vi "Main.vi"() -> ()   [LabVIEW 2013]
uses:
  <vilib>/myRIO/Instrument Drivers/Onboard IO/I2C/vis/Smart Open.vi
  <vilib>/myRIO/Instrument Drivers/Onboard IO/I2C/vis/Configure.vi
  <vilib>/myRIO/Instrument Drivers/Onboard IO/I2C/vis/Write.vi
  <vilib>/myRIO/Common/Instrument Driver Framework/myRIO v1.0/UART/vis/myRIO v1.0 Close UART.vi
  <vilib>/myRIO/Instrument Drivers/Onboard IO/I2C/vis/Open.vi
  <vilib>/myRIO/Common/Instrument Driver Framework/myRIO v1.0/I2C/vis/myRIO v1.1 Open I2C.vi
  <vilib>/myRIO/Common/Instrument Driver Framework/Utilities/vis/Validate Channels.vi
  <vilib>/myRIO/Common/Instrument Driver Framework/myRIO v1.0/I2C/vis/myRIO v1.0 Reserve I2C.vi
  <vilib>/myRIO/Common/Instrument Driver Framework/myRIO v1.0/I2C/vis/myRIO v1.0 Build MUX Configuration I2C.vi
  <vilib>/myRIO/Common/Instrument Driver Framework/myRIO v1.0/Resource Manager/vis/myRIO v1.0 Reserve Channel List.vi
  <vilib>/myRIO/Common/Instrument Driver Framework/myRIO v1.0/Resource Manager/vis/myRIO v1.0 Create Configuration List.vi
  <vilib>/myRIO/Common/Instrument Driver Framework/myRIO v1.0/Resource Manager/vis/myRIO v1.0 Reserve Channel.vi
  <vilib>/myRIO/Common/Instrument Driver Framework/myRIO v1.0/Resource Manager/vis/myRIO v1.0 Unreserve Channel.vi
  <vilib>/myRIO/Common/Instrument Driver Framework/myRIO v1.0/Resource Manager/vis/myRIO v1.0 Build Mutex Name.vi
  <vilib>/Instr/_visa.llb/VISA Configure Serial Port (Instr).vi
  <vilib>/myRIO/Common/Instrument Driver Framework/myRIO v1.0/myRIO v1.1 Open.vi
  <vilib>/Utility/VariantDataType/GetNumericInfo.vi
  <vilib>/Utility/error.llb/Error Cluster From Error Code.vi
  <vilib>/myRIO/Common/Instrument Driver Framework/Utilities/vis/IO Manager.vi
  <vilib>/myRIO/Common/Instrument Driver Framework/Utilities/vis/Configuration Manager.vi
  <vilib>/myRIO/Common/Instrument Driver Framework/myRIO v1.0/Resource Manager/vis/myRIO v1.0 Configure IO.vi
  <vilib>/myRIO/Common/Instrument Driver Framework/myRIO v1.0/myRIO v1.0 Close.vi
  <vilib>/myRIO/Common/Instrument Driver Framework/myRIO v1.0/I2C/vis/myRIO v1.0 Configure I2C.vi
  <vilib>/myRIO/Common/Instrument Driver Framework/myRIO v1.0/I2C/vis/myRIO v1.0 Write I2C.vi
  <vilib>/myRIO/Common/Instrument Driver Framework/Utilities/vis/FPGA Ref Manager.vi
  <vilib>/myRIO/Common/Instrument Driver Framework/myRIO v1.0/myRIO v1.0 Reset FPGA.vi
  <vilib>/myRIO/Instrument Drivers/Utilities/Utilities.lvlib
panel:
  in  "[ESC]":bool
  # "Digital tape measure"
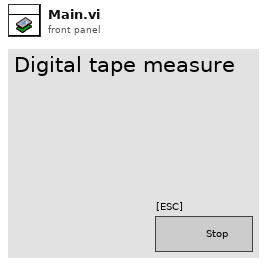
[diagram p1: front panel]
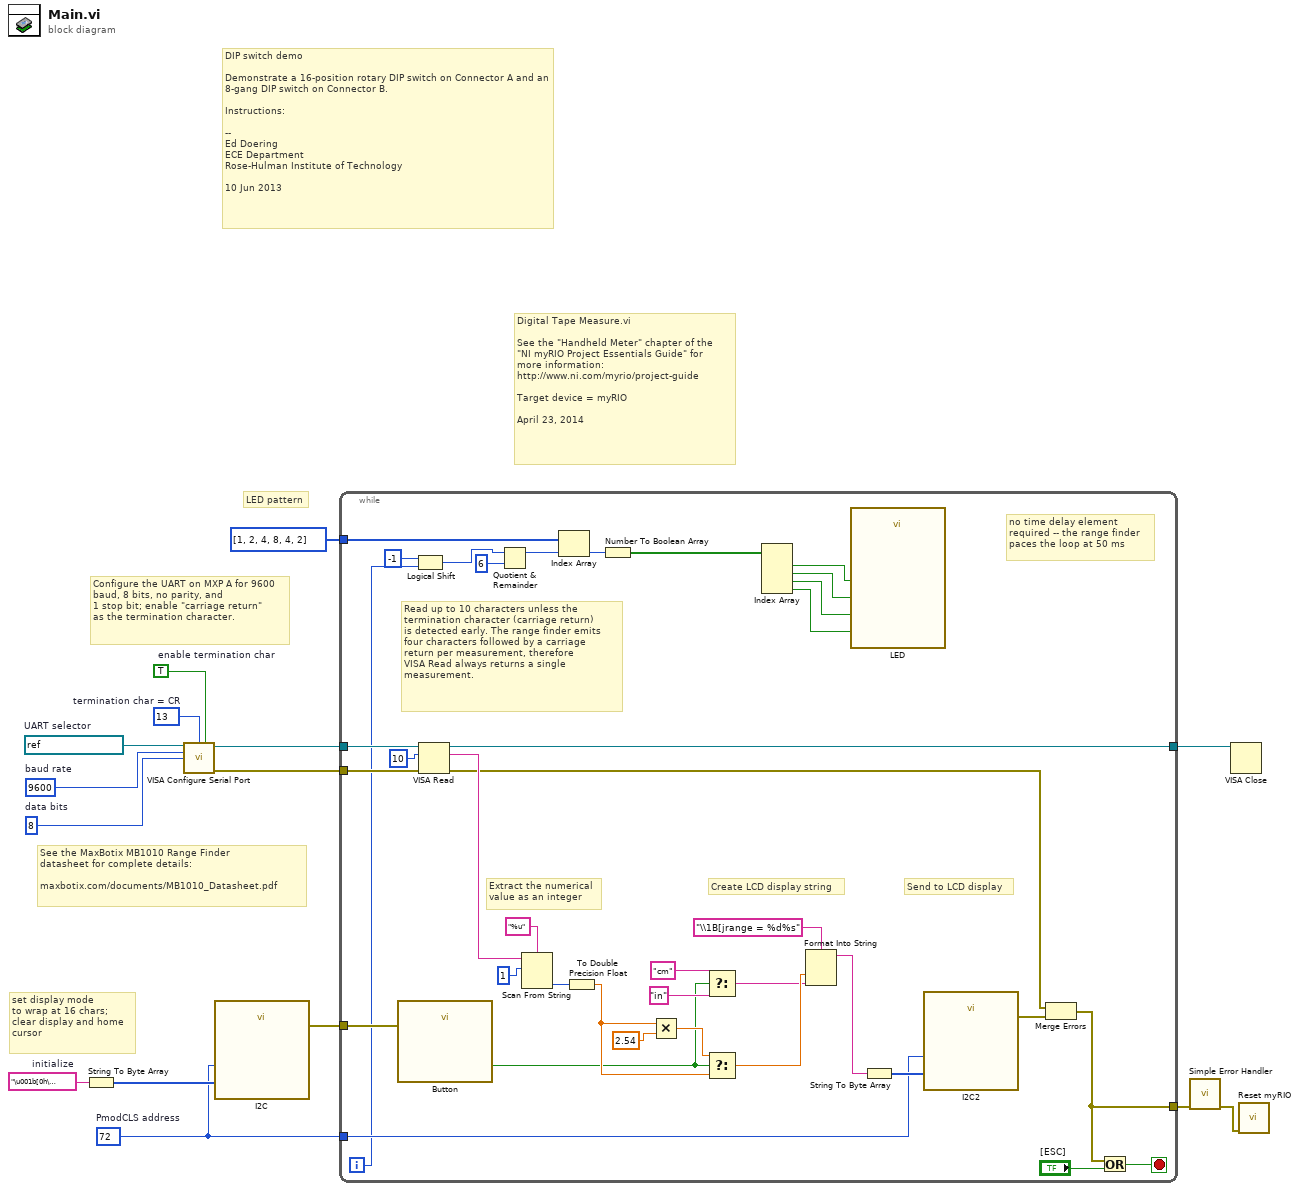
[diagram p0: block diagram]
diagram:
  w5 = u8 13  # termination char = CR
  w9 = refnum<visa-resource-name> "ASRL2::INSTR"  # UART selector
  w6 = TRUE  # enable termination char
  w7 = u16 8  # data bits
  w8 = u32 9600  # baud rate
  w10 = u8 72  # PmodCLS address
  w13 = "\u001b[0h\u001b[j"  # initialize
  # "Digital Tape Measure.vi\n\nSee the \"Handheld Meter\" chapter of the \n\"NI myRIO Project Essentials Guide\" for\nmore information: \nhttp://www.ni.com/myrio/project-guide\n\nTarget device = myRIO\n\nApril 23, 2014"
  # "LED pattern"
  # "See the MaxBotix MB1010 Range Finder\ndatasheet for complete details:\n\nmaxbotix.com/documents/MB1010_Datasheet.pdf"
  # "Configure the UART on MXP A for 9600 baud, 8 bits, no parity, and\n1 stop bit; enable \"carriage return\"\nas the termination character."
  # "set display mode\nto wrap at 16 chars;\nclear display and home\ncursor"
  # "DIP switch demo\n\nDemonstrate a 16-position rotary DIP switch on Connector A and an 8-gang DIP switch on Connector B.\n\nInstructions:\n\n-- \nEd Doering\nECE Department\nRose-Hulman Institute of Technology\n\n10 Jun 2013"
  n1 = String To Byte Array(string=w13) -> (unsigned byte array=w11:u8[])
  n2 = call-poly "VISA Configure Serial Port"("VISA resource name"=w9, "termination char\n(0xA = '\\n' = LF)"=w5, "Enable Termination\nChar (T)"=w6, "baud rate (9600)"=w8, "data bits (8)"=w7) -> ("VISA resource name out"=w4:refnum<visa-resource-name>, "error out"=w3:errorcluster)  [unwired: 9 in]
  n3 = call "I2C"("Slave Address (7-bit)"=w10, "Bytes to Write"=w11) -> ("error out"=w12:errorcluster)  [unwired: 25 in]
  n4 = while {
    tunnel: [w30] -> w14
    tunnel: w12 -> [w41]
    tunnel: w10 -> [w23]
    tunnel: w4 -> [w44]
    tunnel: w3 -> [w43]
    tunnel: [w42] -> w2
    tunnel: u8[] [1, 2, 4, 8, 4, 2] -> [w21]
    i -> [w18]
    stop <- w52 stop-if-true
    # "Send to LCD display"
    # "Create LCD display string"
    # "Read up to 10 characters unless the \ntermination character (carriage return)\nis detected early. The range finder emits\nfour characters followed by a carriage\nreturn per measurement, therefore\nVISA Read always returns a single measurement."
    # "no time delay element\nrequired -- the range finder\npaces the loop at 50 ms"
    # "Extract the numerical\nvalue as an integer"
    n5 = call "Button"("error in (no error)"=w41) -> ("Value"=w34:bool)  [unwired: 25 in, 1 out]
    n6 = Logical Shift(y=i16 -1, x=w18) -> (x << y=w16:i32)
    n7 = VISA Read(VISA resource name=w44, byte count=u32 10, error in (no error)=w43) -> (VISA resource name out=w42:refnum<visa-resource-name>, read buffer=w45:string, error out=w31:errorcluster)  [unwired: 1 out]
    n8 = Quotient & Remainder(x=w16, y=6) -> (x-y*floor(x/y)=w19:i32)  [unwired: 1 out]
    n9 = Scan From String "Scan From String"(format string="%u", input string=w45, initial scan location=u32 1) -> (output 1=w24:u32)  [unwired: 2 in, 3 out]
    n10 = Index Array "Index Array"(array=w21, index=w19) -> (element=w20:u8)
    n11 = To Double Precision Float(number=w24) -> (double precision float=w38:dbl)
    n12 = Number To Boolean Array(number=w20) -> (Boolean array=w29:bool[])
    n13 = Multiply(x=w38, y=2.54) -> (x*y=w39:dbl)
    n14 = Select(t="cm", s=w34, f="in") -> (s? t:f=w33:string)
    n15 = Select(t=w39, s=w34, f=w38) -> (s? t:f=w37:dbl)
    n16 = Index Array(array=w29) -> (element #1=w28:bool, element #2=w27:bool, element #3=w26:bool, element #4=w25:bool)  [unwired: 4 in]
    n17 = Format Into String "Format Into String"(format string="\\1B[jrange = %d%s" ("main display"), w37, w33) -> (resulting string=w50:string)  [unwired: 2 in, 1 out]
    n18 = call "LED"("LED0"=w28, "LED1"=w27, "LED2"=w26, "LED3"=w25) -> ()  [unwired: 23 in, 1 out]
    n19 = String To Byte Array(string=w50) -> (unsigned byte array=w49:u8[])
    n20 = call "I2C2"("Slave Address (7-bit)"=w23, "Bytes to Write"=w49) -> ("error out"=w32:errorcluster)  [unwired: 25 in]
    n21 = Merge Errors(w31, w32) -> (w30:errorcluster)
    n22 = Or(x=w30, y="[ESC]") -> (x .or. y?=w52:bool)
  }
  n23 = call <vilib>:"Simple Error Handler.vi"("error in (no error)"=w14) -> ("error out"=w15:errorcluster)  [unwired: 4 in, 4 out]
  n24 = VISA Close(VISA resource name=w2) -> ()  [unwired: 1 in, 1 out]
  n25 = call <vilib>:"Reset myRIO.vi"("error in (no error)"=w15) -> ()  [unwired: 10 in, 1 out]
